vi "MAX_ASCII.vi"() -> ()   [LabVIEW 2018]
uses:
  <vilib>/Instr/_visa.llb/VISA Configure Serial Port (Instr).vi
panel:
  in  "file path (use dialog)":path
  in  "flow control":u16(ring) items=["None", "XON/XOFF", "RTS/CTS", "XON/XOFF & RTS/CTS", "DTR/DSR", "XON/XOFF & DTR/DSR"]
  in  "parity":enum16{"None", "Odd", "Even", "Mark", "Space"}(ring)
  in  "data bits":u16=8 min=5 max=8 step=1
  in  "baud rate":u32=9600
  in  "stop bits":u16(ring)=10 items=["1.0"=10, "1.5"=15, "2.0"=20]
  out "concatenated string":string
  out "Table of data":string[][](table)
  in  "Start Reading":bool
  in  "Stop Simulation":bool
  in  "Serial Port":refnum<visa-resource-name>
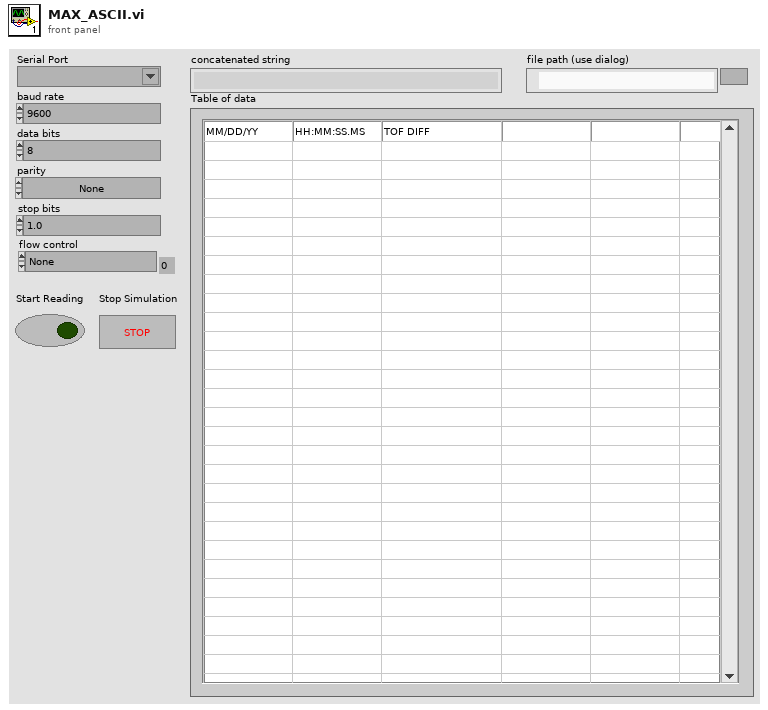
[diagram p1: front panel]
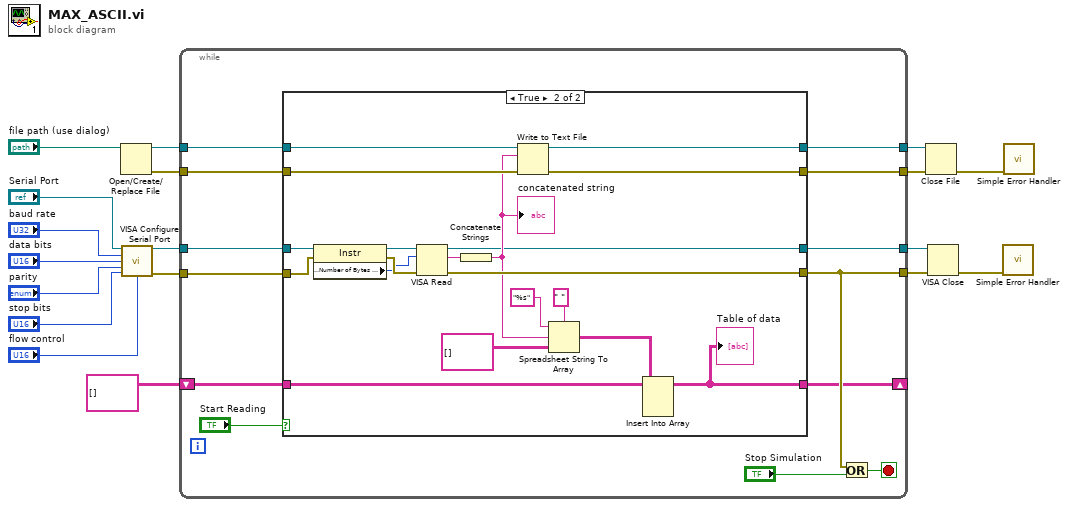
[diagram p0: block diagram]
diagram:
  n1 = Open/Create/Replace File(file path (use dialog)="file path (use dialog)") -> (refnum out=w6:refnum<file>, error out=w7:errorcluster)  [unwired: 5 in, 1 out]
  n2 = call-poly "VISA Configure Serial Port"("VISA resource name"="Serial Port", "baud rate (9600)"="baud rate", "data bits (8)"="data bits", "parity (0:none)"="parity", "stop bits (10: 1 bit)"="stop bits", "flow control (0:none)"="flow control") -> ("VISA resource name out"=w14:refnum<visa-resource-name>, "error out"=w18:errorcluster)  [unwired: 8 in]
  n3 = while {
    tunnel: w18 -> [w31]
    tunnel: [w27] -> w17
    tunnel: [w26] -> w16
    tunnel: w14 -> [w25]
    tunnel: w7 -> [w24]
    tunnel: w6 -> [w23]
    tunnel: [w22] -> w5
    tunnel: [w21] -> w4
    shift-right: [w19] -> _
    shift-left: string[][] [] ("element") -> [w20]
    stop <- w29 stop-if-true
    n4 = case shown="True" "Start Reading" {
      tunnel: w31 -> [w35 w54]
      tunnel: [w35 w55] -> w27
      tunnel: [w36 w40] -> w26
      tunnel: w25 -> [w36 w49]
      tunnel: w24 -> [w34 w44]
      tunnel: w23 -> [w33 w45]
      tunnel: [w33 w43] -> w22
      tunnel: [w34 w42] -> w21
      tunnel: w20 -> [w32 w39]
      tunnel: [w32 w38] -> w19
      frame False {
      }
      frame True {
        n5 = property class="Instr"(reference=w49, error in=w54) -> (reference out=w52:refnum<visa-resource-name>, error out=w53:errorcluster, "Serial Settings:Number of Bytes at Serial Port"=w51:u32)
        n6 = VISA Read(VISA resource name=w52, byte count=w51, error in (no error)=w53) -> (VISA resource name out=w40:refnum<visa-resource-name>, read buffer=w50:string, error out=w55:errorcluster)  [unwired: 1 out]
        n7 = Concatenate Strings(w50) -> (w41:string)
        "concatenated string" <- w41
        n8 = Write to Text File(file (use dialog)=w45, text=w41, error in=w44) -> (refnum out=w43:refnum<file>, error out=w42:errorcluster)  [unwired: 1 in, 1 out]
        n9 = Spreadsheet String To Array(delimiter (Tab)=" ", format string="%s", spreadsheet string=w41, array type (2D Dbl)=string[][] [] ("Array")) -> (array=w37:string[][])
        n10 = Insert Into Array(array=w39, new element=w37) -> (w38:string[][])  [unwired: 2 in]
        "Table of data" <- w38
      }
    }
    n11 = Or(x=w27, y="Stop Simulation") -> (x .or. y?=w29:bool)
  }
  n12 = Close File(refnum=w5, error in=w4) -> (error out=w3:errorcluster)  [unwired: 1 out]
  n13 = VISA Close(VISA resource name=w16, error in (no error)=w17) -> (error out=w13:errorcluster)
  n14 = call <vilib>:"Simple Error Handler.vi"("error in (no error)"=w13) -> ()  [unwired: 4 in, 5 out]
  n15 = call <vilib>:"Simple Error Handler.vi"("error in (no error)"=w3) -> ()  [unwired: 4 in, 5 out]
